vi "GetDLLPath.vi"(9 "VI-Path":path) -> (1 "DLL-Path":path)   [LabVIEW 2015, in "MEDAQLib.lvlib"]
doc: "This VI takes the current VI-Path and returns the path to the MEDAQLib.dll."
uses:
  MEDAQLib.lvlib
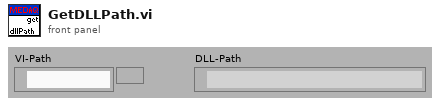
[diagram p1: front panel]
types:
  T1 = enum32{"invalid app kind", "Development System", "Run Time System", "Student Edition", "Embedded LabVIEW", "Evaluation", "Custom"}
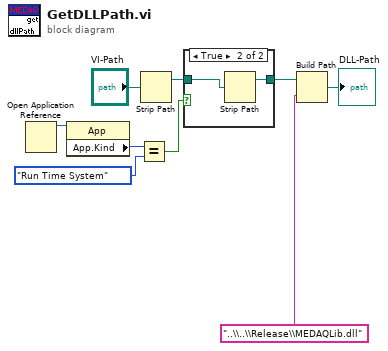
[diagram p0: block diagram]
diagram:
  n1 = Open Application Reference() -> (3:w3:refnum<vi>)  [unwired: 1 in, 4 out]
  n2 = property class="App"(reference=w3) -> ("App.Kind"=w4:T1)  [unwired: 1 in, 2 out]
  n3 = Equal?(x=w4, y=T1."Run Time System" ("Applikation:Typ")) -> (x = y?=w6:bool)
  n4 = Strip Path(path="VI-Path") -> (stripped path=w2:path)  [unwired: 1 out]
  n5 = case shown="True" w6 {
    tunnel: w2 -> [w10 w12]
    tunnel: [w10 w11] -> w7
    frame False {
    }
    frame True {
      n6 = Strip Path(path=w12) -> (stripped path=w11:path)  [unwired: 1 out]
    }
  }
  n7 = Build Path(base path=w7, name or relative path="..\\..\\Release\\MEDAQLib.dll" ("Name oder relativer Pfad")) -> (appended path=→"DLL-Path":path)
